vi "Conn Add Recordset Reference.vi"(8 "error in (no error)":errorcluster, 11 "connection reference":T1) -> (0 "error out":errorcluster)   [LabVIEW 2017, in "NI_Database_API.lvlib"]
doc: "Adds a recordset reference to the specified <B>connection reference</B>."
uses:
  <vilib>/addons/database/NI_Database_API.lvlib
  <vilib>/addons/database/Connection.llb/Conn ObjectReference.ctl
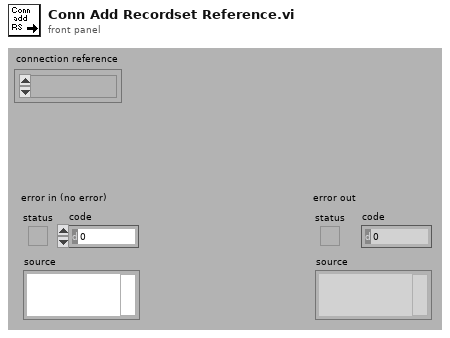
[diagram p1: front panel]
types:
  T1 = typedef "NI_Database_API.lvlib/Conn ObjectReference.ctl" = refnum<k1>
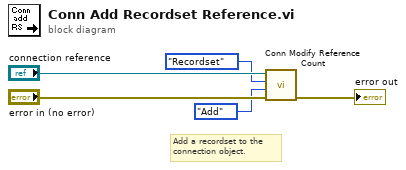
[diagram p0: block diagram]
diagram:
  # "Add a recordset to the\nconnection object."
  n1 = call <vilib>:"Conn Modify Reference Count.vi"("error in (no error)"="error in (no error)", "operation"=enum16{"Add", "Subtract"}."Add" ("Operation"), "object"=enum16{"Recordset", "Command"}."Recordset" ("Object"), "connection reference"="connection reference") -> ("error out"=→"error out":errorcluster)  [unwired: 4 in, 1 out]
